vi "Configure Pulse-Train.vi"(7 "Pulse-Train Data":T1(array[cluster])=[{"Level (1 V)"=1.0, "Width (0.02 s)"=0.02, "Delay (0 s)"=0.0}], 8 "error in (no error)":errorcluster, 9 "Pulse-Train Offset (0 V)":dbl, 10 "Pulse-Train Period (0.025 s)":dbl=0.025, 11 "VISA resource name":refnum<visa-resource-name>) -> (0 "error out":errorcluster, 3 "VISA resource name out":refnum<visa-resource-name>)   [LabVIEW 2015, in "Fluke 28x Series.lvlib"]
doc: "Configures a series of pulses which make up the pulse-train. This is one of the standard waveforms that can be output by the generator."
uses:
  <instrlib>/Fluke 28x Series/Fluke 28x Series.lvlib
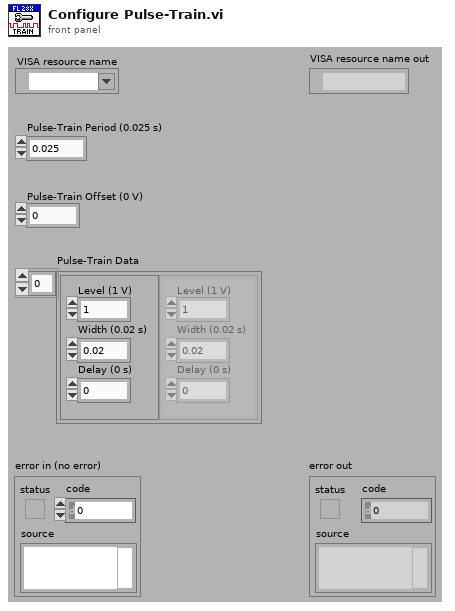
[diagram p1: front panel]
types:
  T1 = cluster{"Level (1 V)":dbl, "Width (0.02 s)":dbl, "Delay (0 s)":dbl}[]
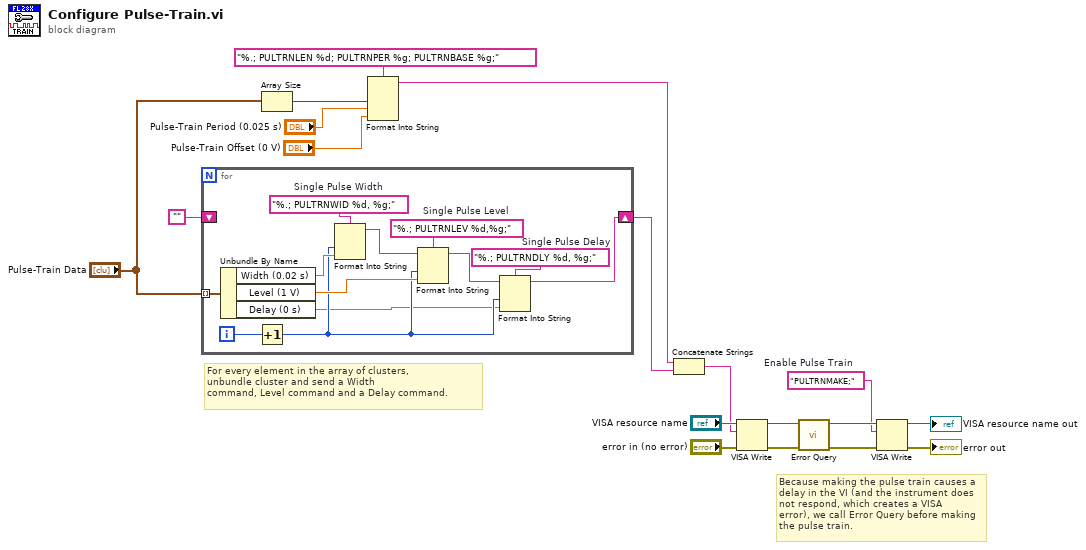
[diagram p0: block diagram]
diagram:
  w5 = "PULTRNMAKE;"  # Enable Pulse Train
  # "Because making the pulse train causes a\ndelay in the VI (and the instrument does \nnot respond, which creates a VISA \nerror), we call Error Query before making\nthe pulse train."
  # "For every element in the array of clusters,\nunbundle cluster and send a Width\ncommand, Level command and a Delay command."
  n1 = for {
    shift-right: [w25] -> w17
    shift-left: "" ("Empty String Constant") -> [_]
    tunnel: "Pulse-Train Data" -> [w19] mode=indexing
    i -> [w30]
    w26 = "%.; PULTRNDLY %d, %g;"  # Single Pulse Delay
    w27 = "%.; PULTRNLEV %d,%g;"  # Single Pulse Level
    w29 = "%.; PULTRNWID %d, %g;"  # Single Pulse Width
    n2 = Unbundle By Name(w19) -> ("Width (0.02 s)"=w28:dbl, "Level (1 V)"=w22:dbl, "Delay (0 s)"=w20:dbl)
    n3 = Increment(x=w30) -> (x+1=w21:i32)
    n4 = Format Into String(format string=w29, w21, w28) -> (resulting string=w23:string)  [unwired: 2 in, 1 out]
    n5 = Format Into String(format string=w27, initial string=w23, w21, w22) -> (resulting string=w24:string)  [unwired: 1 in, 1 out]
    n6 = Format Into String(format string=w26, initial string=w24, w21, w20) -> (resulting string=w25:string)  [unwired: 1 in, 1 out]
  }
  n7 = Array Size(array="Pulse-Train Data") -> (size(s)=w10:i32)
  n8 = Format Into String(format string="%.; PULTRNLEN %d; PULTRNPER %g; PULTRNBASE %g;", w10, "Pulse-Train Period (0.025 s)", "Pulse-Train Offset (0 V)") -> (resulting string=w3:string)  [unwired: 2 in, 1 out]
  n9 = Concatenate Strings(w3, w17) -> (w15:string)
  n10 = VISA Write(VISA resource name="VISA resource name", write buffer=w15, error in (no error)="error in (no error)") -> (VISA resource name out=w9:refnum<visa-resource-name>, error out=w8:errorcluster)  [unwired: 1 out]
  n11 = call <instrlib>:"Error Query.vi"("error in (no error)"=w8, "VISA resource name"=w9) -> ("error out"=w6:errorcluster, "VISA resource name out"=w7:refnum<visa-resource-name>)  [unwired: 6 in, 2 out]
  n12 = VISA Write(VISA resource name=w7, write buffer=w5, error in (no error)=w6) -> (VISA resource name out=→"VISA resource name out":refnum<visa-resource-name>, error out=→"error out":errorcluster)  [unwired: 1 out]
